vi "Discover Devices.vi"(2 "error in (no error)":errorcluster) -> (0 "error out":errorcluster, 1 "Devices":T1[](array[typedef]))   [LabVIEW 2010]
uses:
  Controls/SpiDevice.ctl
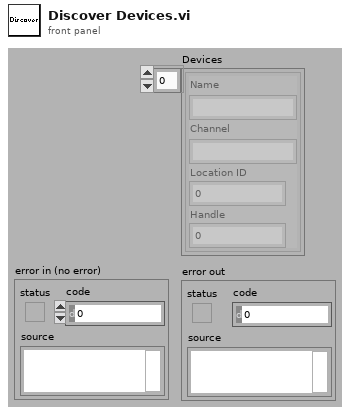
[diagram p1: front panel]
types:
  T1 = typedef "SpiDevice.ctl" = cluster{"Name":string, "Channel":string, "Location ID":u32, "Handle":u32}
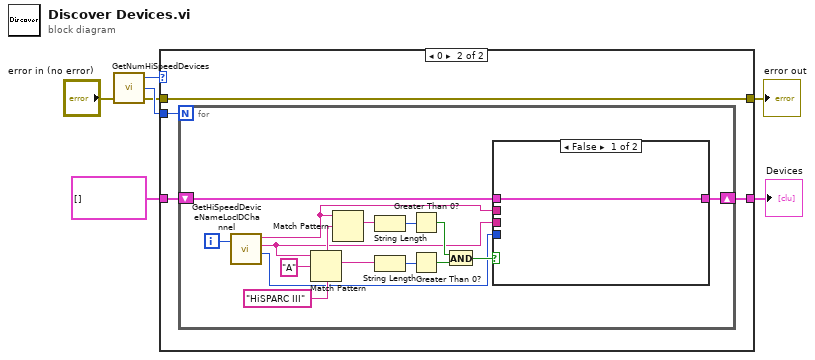
[diagram p0: block diagram]
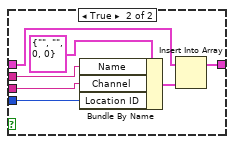
[diagram p3: hidden frame]
diagram:
  n1 = call "GetNumHiSpeedDevices.vi"("error in (no error)"="error in (no error)") -> ("error out"=w4:errorcluster, "device count"=w6:u32, "result"=w5:u32)  [unwired: 2 in]
  n2 = case shown="0" w5 {
    tunnel: w6 -> [_ w13]
    tunnel: w4 -> [w8 w12]
    tunnel: [w8 w12] -> w1
    tunnel: T1[] [] -> [w9 w11]
    tunnel: [w9 w10] -> w2
    frame Default {
    }
    frame 0 {
      n3 = for {
        N: w13 -> [_]
        shift-right: [w14] -> w10
        shift-left: w11 -> [w15]
        i -> [w28]
        n4 = call "GetHiSpeedDeviceNameLocIDChannel.vi"("Device index"=w28) -> ("Device name"=w18:string, "Device channel"=w17:string, "Location ID"=w16:u32)  [unwired: 1 in, 1 out]
        n5 = Match Pattern(string=w17, regular expression="A") -> (match substring=w24:string)  [unwired: 1 in, 3 out]
        n6 = Match Pattern(string=w18, regular expression="HiSPARC III") -> (match substring=w25:string)  [unwired: 1 in, 3 out]
        n7 = String Length(string=w25) -> (length=w23:i32)
        n8 = String Length(string=w24) -> (length=w22:i32)
        n9 = Greater Than 0?(x=w23) -> (x > 0?=w20:bool)
        n10 = Greater Than 0?(x=w22) -> (x > 0?=w21:bool)
        n11 = And(x=w20, y=w21) -> (x .and. y?=w19:bool)
        n12 = case shown="False" w19 {
          tunnel: w18 -> [_ w35]
          tunnel: w17 -> [_ w34]
          tunnel: w16 -> [_ w33]
          tunnel: w15 -> [w29 w32]
          tunnel: [w29 w31] -> w14
          frame False {
          }
          frame True {
            n13 = Bundle By Name(cluster=T1 {"Name"="", "Channel"="", "Location ID"=0, "Handle"=0} ("SPI Device"), "Name"=w35, "Channel"=w34, "Location ID"=w33) -> (w30:T1)
            n14 = Insert Into Array(array=w32, new element=w30) -> (w31:T1[])  [unwired: 1 in]
          }
        }
      }
    }
  }
  "Devices" <- w2
  "error out" <- w1
